vi "Read Run.vi"(8 "error in (no error)":errorcluster, 11 "MB in":refnum<class "Modbus Master CR.lvclass">) -> (0 "error out":errorcluster, 2 "Run":bool, 3 "MB out":refnum<class "Modbus Master CR.lvclass">)   [LabVIEW 2021, in "Modbus Master CR.lvclass"]
uses:
  Modbus Master CR.lvclass
  Modbus Master CR.lvclass/Modbus Master CR.ctl
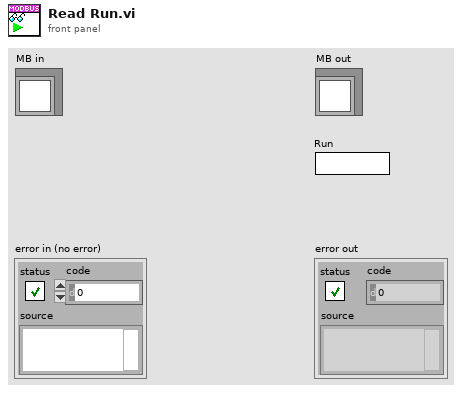
[diagram p1: front panel]
types:
  T1 = typedef "Modbus Master CR.lvclass/MB state.ctl" = cluster{"state":T2, "enable":bool, "Run":bool, "write enable":bool, "Write":bool, "connect":bool, "errors":i32}
  T2 = typedef "MB_v2.lvlib/Modbus Master CR.lvclass/MB_TCP_State.ctl" = enum8{"initialization", "redefine", "standby", "ping", "connect", "wait to reconnect", "wait to reset timeout", "configure", "requests", "close connection", "stop"}
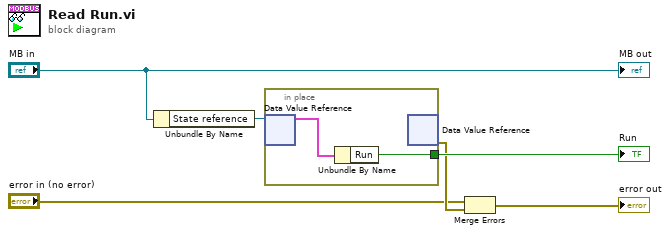
[diagram p0: block diagram]
diagram:
  n1 = Unbundle By Name("MB in") -> ("State reference"=w3:refnum<data-value>)
  n2 = in-place {
    in-place-border: [w8] -> w4
    n3 = in-place-dvr #1(w3) -> (w7:T1)  [unwired: 1 out]
    n4 = Unbundle By Name(w7) -> ("Run"=w8:bool)
    n5 = in-place-dvr #1() -> (w2:errorcluster)  [unwired: 1 in, 1 out]
  }
  "Run" <- w4
  n6 = Merge Errors("error in (no error)", w2) -> (→"error out":errorcluster)
  "MB out" <- "MB in"
